vi "Find_ThresholdOphir_F4.vi"(5 "Threshold Ophir":dbl, 8 "Current array":dbl[](array[numeric]), 11 "Ophir array":dbl[](array[numeric])) -> (2 "Threshold Current":dbl)   [LabVIEW 2013]
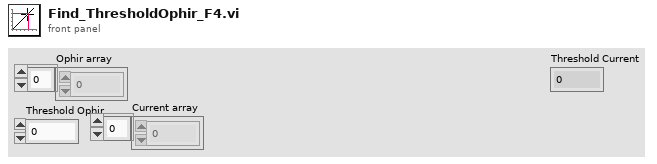
[diagram p1: front panel]
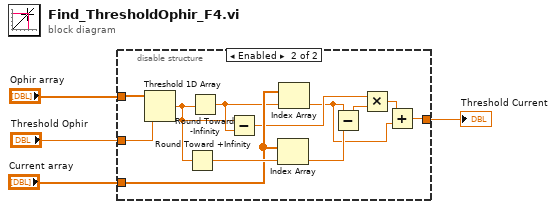
[diagram p0: block diagram]
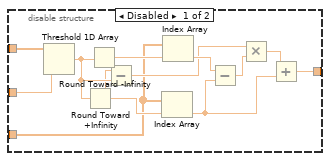
[diagram p2: hidden frame]
diagram:
  n1 = disable-structure shown="Enabled" {
    disable-tunnel: "Ophir array" -> [w8 w25]
    disable-tunnel: "Threshold Ophir" -> [w7 w24]
    disable-tunnel: "Current array" -> [w6 w23]
    disable-tunnel: [w5 w22] -> w1
    frame Disabled {
      n2 = Threshold 1D Array(2:w7, 3:w8) -> (0:w16:dbl)  [unwired: 1 in]
      n3 = Round Toward +Infinity(x=w16) -> (ceil(x): smallest int >= x=w14:dbl)
      n4 = Round Toward -Infinity(1:w16) -> (0:w15:dbl)
      n5 = Subtract(x=w14, y=w16) -> (x-y=w11:dbl)
      n6 = Index Array(array=w6, index=w14) -> (element=w9:dbl)
      n7 = Index Array(array=w6, index=w15) -> (element=w13:dbl)
      n8 = Subtract(x=w13, y=w9) -> (x-y=w12:dbl)
      n9 = Multiply(x=w11, y=w12) -> (x*y=w10:dbl)
      n10 = Add(x=w10, y=w9) -> (x+y=w5:dbl)
    }
    frame Enabled {
      n11 = Threshold 1D Array(2:w24, 3:w25) -> (0:w20:dbl)  [unwired: 1 in]
      n12 = Round Toward +Infinity(x=w20) -> (ceil(x): smallest int >= x=w28:dbl)
      n13 = Round Toward -Infinity(1:w20) -> (0:w21:dbl)
      n14 = Subtract(x=w20, y=w21) -> (x-y=w18:dbl)
      n15 = Index Array(array=w23, index=w28) -> (element=w19:dbl)
      n16 = Index Array(array=w23, index=w21) -> (element=w17:dbl)
      n17 = Subtract(x=w17, y=w19) -> (x-y=w27:dbl)
      n18 = Multiply(x=w18, y=w27) -> (x*y=w26:dbl)
      n19 = Add(x=w26, y=w17) -> (x+y=w22:dbl)
    }
  }
  "Threshold Current" <- w1
